vi "DefendGoalTacticCheckStateChange.vi"(8 "error in (no error)":errorcluster, 10 "Game":refnum<class "Game.lvclass">, 11 "DefendGoalTactic in":refnum<class "DefendGoalTactic.lvclass">) -> (0 "error out":errorcluster, 2 "States":T1, 3 "DefendGoalTactic out":refnum<class "DefendGoalTactic.lvclass">)   [LabVIEW 2024, in "DefendGoalTactic.lvclass"]
uses:
  DefendGoalTactic.lvclass
  Game_class/Game.lvclass
  DefendGoalTacticStates.ctl
  Referee_class/command_interpreted.ctl
  Game_class/Game.lvclass/Game.ctl
  Referee_class/Referee.lvclass/Referee.ctl
  Object_class/Object.lvclass/Object.ctl
  Parameters_class/Parameters.lvclass/Parameters.ctl
  Team_class/Team.lvclass/Team.ctl
  Ball_class/Ball.lvclass/Ball.ctl
  Team_class/Read RobotRef.vi
  Game_class/Read FieldRef.vi
  Game_class/Read Referee.vi
  Game_class/Read OffensiveTeam.vi
  Game_class/Read Utilities.lvclass.vi
  Game_class/Read EnemyRef.vi
  Game_class/Read BallRef.vi
  Game_class/Read Parameters.lvclass.vi
  Parameters_class/Read AttakingOurselves.vi
  Object_class/Read position(x,y).vi
  Ball_class/Read velocityNorm.vi
  Referee_class/Read command_interpreted.vi
  <vilib>/Analysis/_algsub.llb/Vector Norm.vi
  <vilib>/Analysis/_algsub.llb/Real Vector Norm.vi
  Ball_class/Ball.lvclass
  C:/Users/as119/OneDrive/Documentos/roboIME/SSL_AI/Object_class/Object.lvclass
  Enemy_class/Enemy.lvclass
  C:/Users/as119/OneDrive/Documentos/roboIME/SSL_AI/Team_class/Team.lvclass
  Ally_class/Ally.lvclass
  Field_class/Field.lvclass
  Referee_class/Referee.lvclass
  Utilities_class/Utilities.lvclass
  Parameters_class/Parameters.lvclass
  Robot_class/Robot.lvclass
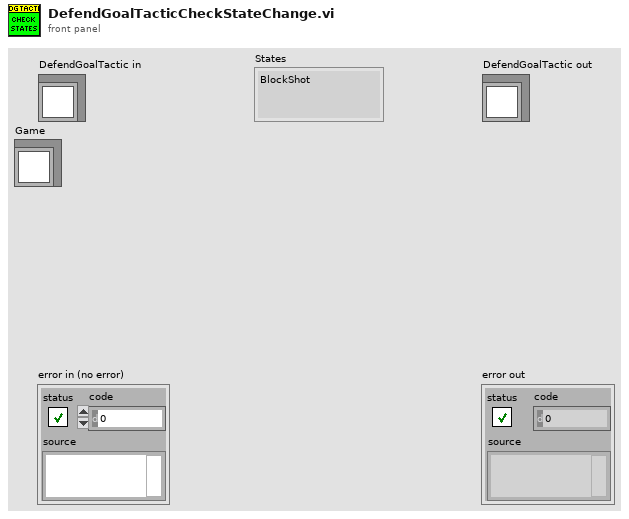
[diagram p1: front panel]
types:
  T1 = typedef "DefendGoalTactic.lvclass/DefendGoalTacticStates.ctl" = enum16{"BlockShot", "BlockPossibleShot", "CoverOneTouchShot", "Kick", "GuardGoal", "Exit", "IsPenalty"}
  T2 = typedef "command_interpreted.ctl" = enum16{"Goal Ally", "Goal Enemy", "Ball Placement Enemy", "Ball Placement Ally", "Normal Half Time", "Extra Time  Break", "Extra Half Time", "None", "Post Game", "PKA Normal Start", "Prepare Kickoff Ally", "PKE Normal Start", "Prepare Kickoff Enemy", "Force Start", "Halt", "Timeout", "Prepare Penalty Ally", "Prepare Penalty Enemy", "PPA NormalStart", "PPE Normal Start", "Indirect Free Ally", "Direct Free Enemy", "Direct Free Ally", "Indirect Free Enemy", "Stop"}
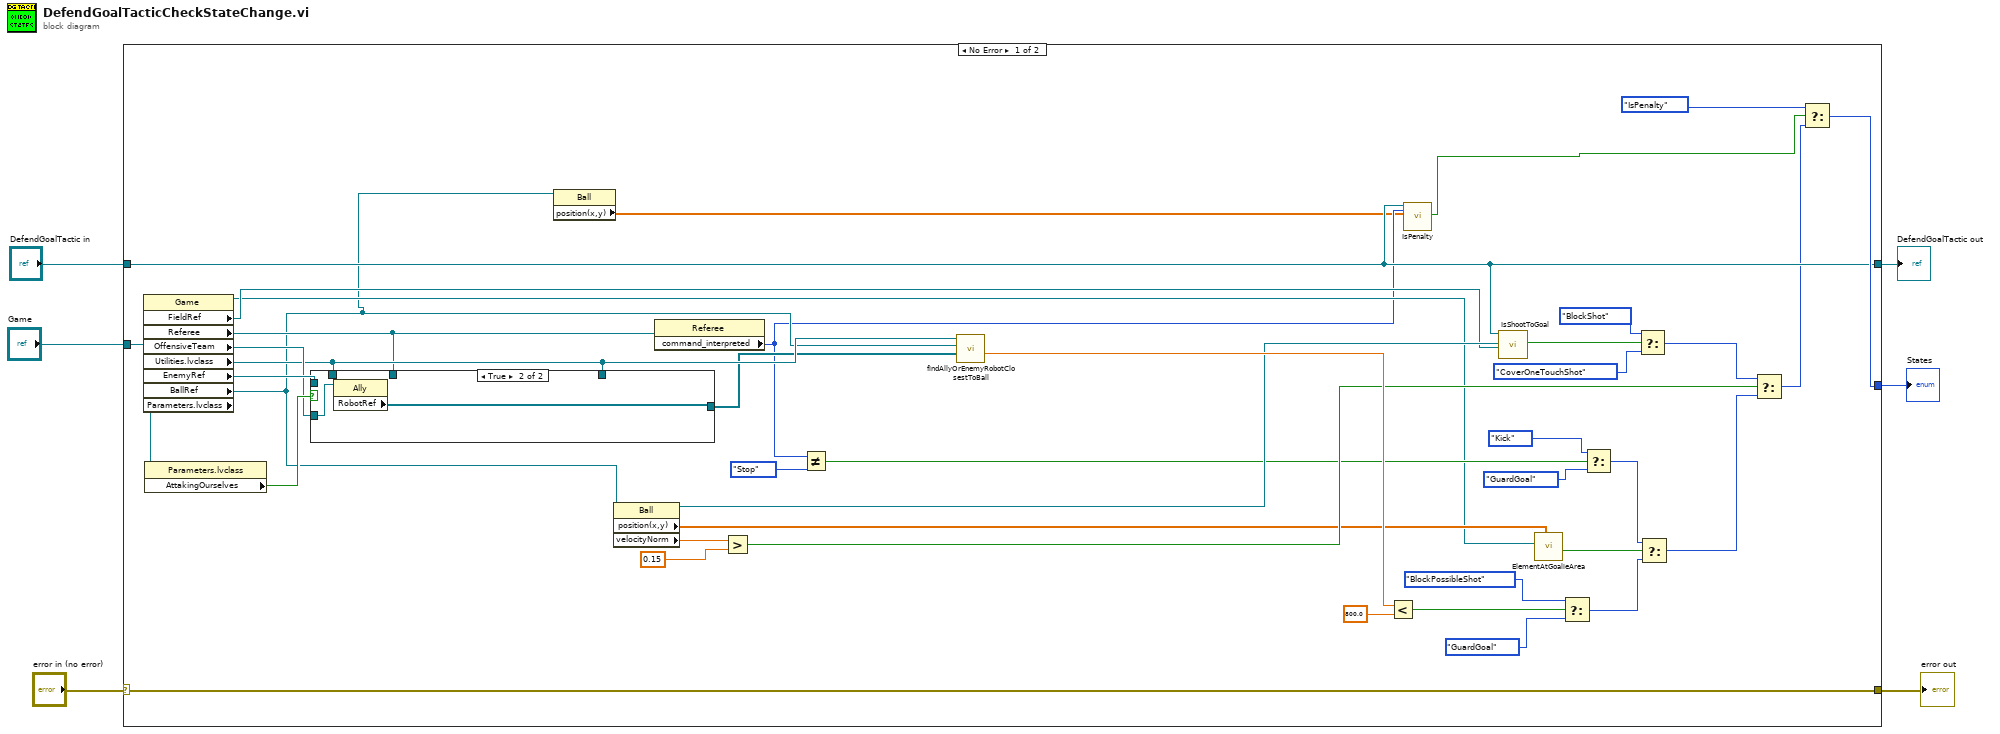
[diagram p0: block diagram]
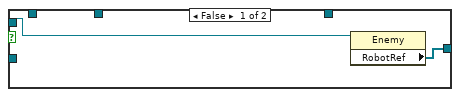
[diagram p2: hidden frame]
diagram:
  n1 = case shown="No Error" "error in (no error)" {
    selector: "error in (no error)" -> [w47 w53]
    tunnel: [w47 w53] -> w5
    tunnel: [w13 w52] -> w3
    tunnel: "DefendGoalTactic in" -> [w13 w52]
    tunnel: "Game" -> [w41 _]
    tunnel: [w14 _] -> w1
    frame No Error {
      n2 = property class="Game"(reference=w41) -> (reference out=w17:refnum<class "Game.lvclass">, "FieldRef"=w30:refnum<class "Field.lvclass">, "Referee"=w40:refnum<class "Referee.lvclass">, "OffensiveTeam"=w44:refnum<class "Ally.lvclass">, "Utilities.lvclass"=w42:refnum<class "Utilities.lvclass">, "EnemyRef"=w46:refnum<class "Enemy.lvclass">, "BallRef"=w10:refnum<class "Ball.lvclass">, "Parameters.lvclass"=w43:refnum<class "Parameters.lvclass">)  [unwired: 1 in, 1 out]
      n3 = property class="Parameters.lvclass"(reference=w43) -> ("AttakingOurselves"=w45:bool)  [unwired: 1 in, 2 out]
      n4 = case shown="True" w45 {
        tunnel: w46 -> [w49 _]
        tunnel: [w48 w50] -> w36
        tunnel: w44 -> [_ w51]
        tunnel: w42 -> [_ _]
        tunnel: w42 -> [_ _]
        tunnel: w40 -> [_ _]
        frame False {
          n5 = property class="Enemy"(reference=w49) -> ("RobotRef"=w48:refnum<class "Robot.lvclass">[])  [unwired: 1 in, 2 out]
        }
        frame True {
          n6 = property class="Ally"(reference=w51) -> ("RobotRef"=w50:refnum<class "Robot.lvclass">[])  [unwired: 1 in, 2 out]
        }
      }
      n7 = property class="Ball"(reference=w10) -> ("position(x,y)"=w8:dbl[])  [unwired: 1 in, 2 out]
      n8 = property class="Ball"(reference=w10) -> (reference out=w31:refnum<class "Ball.lvclass">, "position(x,y)"=w27:dbl[], "velocityNorm"=w35:dbl)  [unwired: 1 in, 1 out]
      n9 = property class="Referee"(reference=w40) -> ("command_interpreted"=w9:T2)  [unwired: 1 in, 2 out]
      n10 = Greater?(x=w35, y=0.15) -> (0:w34:bool)
      n11 = Not Equal?(x=w9, y=command_interpreted."Stop") -> (x != y?=w19:bool)
      n12 = call "findAllyOrEnemyRobotClosestToBall.vi"("Ally/Enemy Robots"=w36, "Ball"=w10, "Utilities in"=w42) -> ("Robot distance to ball"=w38:dbl)  [unwired: 4 in, 4 out]
      n13 = Less?(x=w38, y=800.0) -> (x < y?=w15:bool)
      n14 = call "IsPenalty.vi"("object in"=w13, "command_interpreted"=w9, "pos(x, y) da bola"=w8) -> ("IsPenalty"=w7:bool)  [unwired: 14 in, 2 out]
      n15 = call "IsShootToGoal.vi"("object in"=w13, "Ball"=w31, "Field"=w30) -> ("IsShoot"=w33:bool)  [unwired: 13 in, 3 out]
      n16 = call "ElementAtGoalieArea.vi"("Elemento pos."=w27, "Game"=w17) -> ("Element at our goalkeeper area ?"=w26:bool)  [unwired: 5 in, 4 out]
      n17 = Select(t=DefendGoalTacticStates."BlockPossibleShot" ("f"), s=w15, f=DefendGoalTacticStates."GuardGoal") -> (s? t:f=w24:T1)
      n18 = Select(t=DefendGoalTacticStates."Kick" ("f"), s=w19, f=DefendGoalTacticStates."GuardGoal") -> (s? t:f=w20:T1)
      n19 = Select(t=DefendGoalTacticStates."BlockShot" ("States"), s=w33, f=DefendGoalTacticStates."CoverOneTouchShot") -> (s? t:f=w32:T1)
      n20 = Select(t=w20, s=w26, f=w24) -> (s? t:f=w25:T1)
      n21 = Select(t=w32, s=w34, f=w25) -> (s? t:f=w11:T1)
      n22 = Select(t=DefendGoalTacticStates."IsPenalty" ("States"), s=w7, f=w11) -> (s? t:f=w14:T1)
    }
    frame Error {
    }
  }
  "error out" <- w5
  "DefendGoalTactic out" <- w3
  "States" <- w1
